vi "保存模拟数据子程序.vi"(0 "Input":T1={"Digital Start Trigger Source 4"="/Dev1/PFI0", "Digital Start Trigger Edge 4"=10280, "minimum value"=-10.0, "maximum value"=10.0, "rate"=1000.0, "device name"="PXI1Slot5", "formular in"=[], "Total time"=0.0} {"rate" format="%0.2f"; "maximum value" format="%0.2f"; "minimum value" format="%0.2f"; "Digital Start Trigger Edge 4" items=["Rising"=10280, "Falling"=10171]}) -> ()   [LabVIEW 2021]
uses:
  <vilib>/Utility/file.llb/Write Delimited Spreadsheet (string).vi
panel:
  # "1、formular in 中sample为各个分段函数的持续时间。\n2、Total time 为总时间，必须大于sample加起来的值。\n3、minimum value和maximum value默认±10V不改。\n4、rate为采样率，即时钟频率\n5、device name为选择的板卡名字，可选为PXI1Slot5-7\n6、Source 为接受触发的端口，Edge为选择上升沿触发\n还是其他类型触发。"
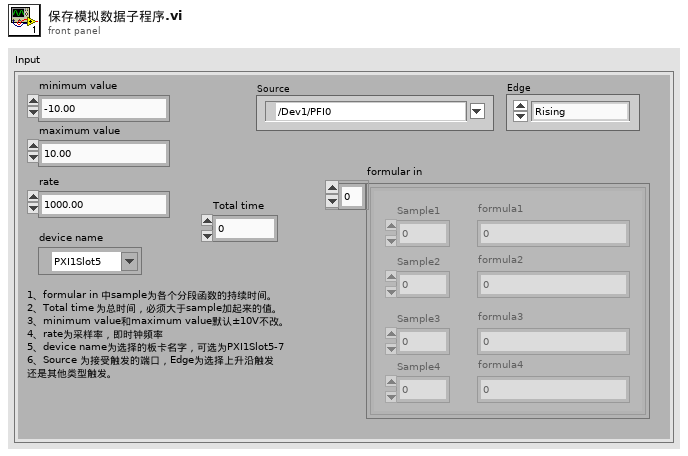
[diagram p1: front panel]
types:
  T1 = cluster{"Digital Start Trigger Source 4":tag, "Digital Start Trigger Edge 4":i32, "minimum value":dbl, "maximum value":dbl, "rate":dbl, "device name":tag, "formular in":cluster{"Sample1":dbl, "formula1":string, "Sample2":dbl, "formula2":string, "Sample3":dbl, "formula3":string, "Sample4":dbl, "formula4":string}[], "Total time":dbl}
  T2 = cluster{"Sample1":dbl, "formula1":string, "Sample2":dbl, "formula2":string, "Sample3":dbl, "formula3":string, "Sample4":dbl, "formula4":string}[]
  T3 = cluster{"formular in[0]":cluster{"Sample1":dbl, "formula1":string, "Sample2":dbl, "formula2":string, "Sample3":dbl, "formula3":string, "Sample4":dbl, "formula4":string}, "formular in[1]":cluster{"Sample1":dbl, "formula1":string, "Sample2":dbl, "formula2":string, "Sample3":dbl, "formula3":string, "Sample4":dbl, "formula4":string}, "formular in[2]":cluster{"Sample1":dbl, "formula1":string, "Sample2":dbl, "formula2":string, "Sample3":dbl, "formula3":string, "Sample4":dbl, "formula4":string}, "formular in[3]":cluster{"Sample1":dbl, "formula1":string, "Sample2":dbl, "formula2":string, "Sample3":dbl, "formula3":string, "Sample4":dbl, "formula4":string}, "formular in[4]":cluster{"Sample1":dbl, "formula1":string, "Sample2":dbl, "formula2":string, "Sample3":dbl, "formula3":string, "Sample4":dbl, "formula4":string}, "formular in[5]":cluster{"Sample1":dbl, "formula1":string, "Sample2":dbl, "formula2":string, "Sample3":dbl, "formula3":string, "Sample4":dbl, "formula4":string}, "formular in[6]":cluster{"Sample1":dbl, "formula1":string, "Sample2":dbl, "formula2":string, "Sample3":dbl, "formula3":string, "Sample4":dbl, "formula4":string}, "formular in[7]":cluster{"Sample1":dbl, "formula1":string, "Sample2":dbl, "formula2":string, "Sample3":dbl, "formula3":string, "Sample4":dbl, "formula4":string}, "formular in[8]":cluster{"Sample1":dbl, "formula1":string, "Sample2":dbl, "formula2":string, "Sample3":dbl, "formula3":string, "Sample4":dbl, "formula4":string}}
  T4 = cluster{"Sample1":dbl, "formula1":string, "Sample2":dbl, "formula2":string, "Sample3":dbl, "formula3":string, "Sample4":dbl, "formula4":string}
  T5 = cluster{"sample 1":string, "formula1":string, "sample 2":string, "formula2":string, "sample 3":string, "formula3":string, "sample 4":string, "formula4":string}
  T6 = cluster{"formula1":string, "formula1":string, "formula1":string, "formula1":string, "formula1":string, "formula1":string, "formula1":string, "formula1":string}
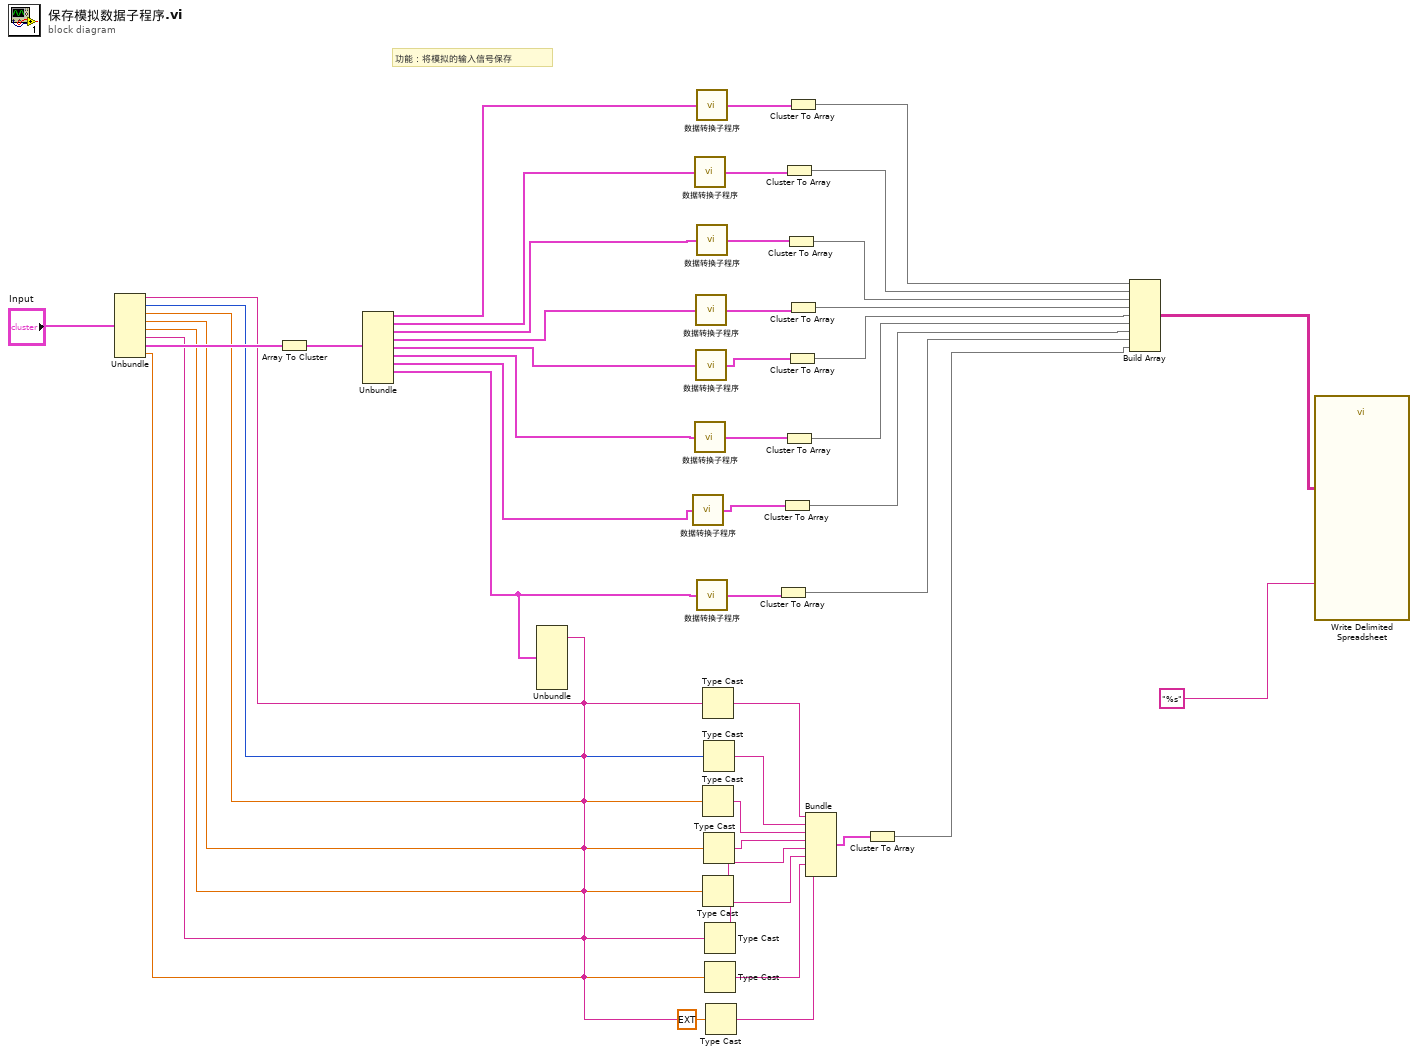
[diagram p0: block diagram]
diagram:
  # "功能：将模拟的输入信号保存"
  n1 = Unbundle("Input") -> ("Digital Start Trigger Source 4"=w30:tag, "Digital Start Trigger Edge 4"=w28:i32, "minimum value"=w27:dbl, "maximum value"=w26:dbl, "rate"=w25:dbl, "device name"=w23:tag, "formular in"=w47:T2, "Total time"=w22:dbl)
  n2 = Array To Cluster(array=w47) -> (cluster=w46:T3)
  n3 = Unbundle(w46) -> ("formular in[0]"=w45:T4, "formular in[1]"=w44:T4, "formular in[2]"=w43:T4, "formular in[3]"=w42:T4, "formular in[4]"=w41:T4, "formular in[5]"=w40:T4, "formular in[6]"=w39:T4, "formular in[7]"=w29:T4)  [unwired: 1 out]
  n4 = Unbundle(w29) -> ("formula1"=w20:string)  [unwired: 7 out]
  n5 = call "数据转换子程序.vi"("formular in[0]"=w39) -> ("output cluster"=w32:T5)
  n6 = call "数据转换子程序.vi"("formular in[0]"=w44) -> ("output cluster"=w37:T5)
  n7 = call "数据转换子程序.vi"("formular in[0]"=w40) -> ("output cluster"=w33:T5)
  n8 = call "数据转换子程序.vi"("formular in[0]"=w42) -> ("output cluster"=w35:T5)
  n9 = call "数据转换子程序.vi"("formular in[0]"=w41) -> ("output cluster"=w34:T5)
  n10 = call "数据转换子程序.vi"("formular in[0]"=w45) -> ("output cluster"=w38:T5)
  n11 = call "数据转换子程序.vi"("formular in[0]"=w43) -> ("output cluster"=w36:T5)
  n12 = call "数据转换子程序.vi"("formular in[0]"=w29) -> ("output cluster"=w31:T5)
  n13 = Type Cast(type=w20, x=w30) -> (*(type *) &x=w19:string)
  n14 = Type Cast(type=w20, x=w27) -> (*(type *) &x=w17:string)
  n15 = Type Cast(type=w20, x=w25) -> (*(type *) &x=w15:string)
  n16 = Type Cast(type=w20, x=w28) -> (*(type *) &x=w18:string)
  n17 = Type Cast(type=w20, x=w26) -> (*(type *) &x=w16:string)
  n18 = Type Cast(type=w20, x=w23) -> (*(type *) &x=w14:string)
  n19 = Type Cast(type=w20, x=w22) -> (*(type *) &x=w13:string)
  n20 = Type Cast(type=w20, x=ext 0.0) -> (*(type *) &x=w12:string)
  n21 = Cluster To Array(cluster=w31) -> (array=w3:string[])
  n22 = Cluster To Array(cluster=w32) -> (array=w4:string[])
  n23 = Cluster To Array(cluster=w37) -> (array=w9:string[])
  n24 = Cluster To Array(cluster=w33) -> (array=w5:string[])
  n25 = Cluster To Array(cluster=w36) -> (array=w8:string[])
  n26 = Cluster To Array(cluster=w34) -> (array=w6:string[])
  n27 = Cluster To Array(cluster=w38) -> (array=w10:string[])
  n28 = Cluster To Array(cluster=w35) -> (array=w7:string[])
  n29 = Bundle("formula1"=w19, "formula1"=w18, "formula1"=w17, "formula1"=w16, "formula1"=w15, "formula1"=w14, "formula1"=w13, "formula1"=w12) -> (w11:T6)  [unwired: 1 in]
  n30 = Cluster To Array(cluster=w11) -> (array=w2:string[])
  n31 = Build Array(w10, w9, w8, w7, w6, w5, w4, w3, w2) -> (w1:string[][])
  n32 = call-poly <vilib>:"Write Delimited Spreadsheet.vi"("format (%s)"="%s" ("format (%.3f)"), "2D data"=w1) -> ()  [unwired: 12 in, 2 out]
